vi "Destroy to Known Hosts.vi"(8 "Error In":errorcluster, 10 "Known Host":refnum<class "Known Host.lvclass">, 11 "Known Hosts In":refnum<class "Known Hosts.lvclass">) -> (0 "Error Out":errorcluster, 3 "Known Hosts Out":refnum<class "Known Hosts.lvclass">)   [LabVIEW 2018, in "Toolkit.lvlib" / "Known Host.lvclass"]
doc: "Passes through the Known Hosts object and destroys the associated Known Host object."
uses:
  Known Host.lvclass
  Known Hosts/Known Hosts.lvclass
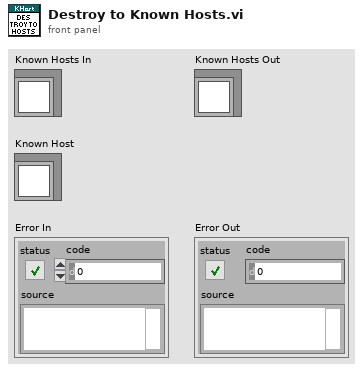
[diagram p1: front panel]
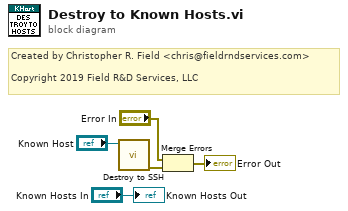
[diagram p0: block diagram]
diagram:
  # "Created by Christopher R. Field <chris@fieldrndservices.com>\n\nCopyright 2019 Field R&D Services, LLC"
  n1 = call "Destroy to SSH.vi"("Known Host"="Known Host") -> ("Error Out"=w2:errorcluster)  [unwired: 9 in, 1 out]
  n2 = Merge Errors("Error In", w2) -> (→"Error Out":errorcluster)
  "Known Hosts Out" <- "Known Hosts In"
